vi "I-V.MODEL.vi"(3 "output control":T1, 4 "data":T2, 5 "x":dbl[](array[numeric]), 6 "a":dbl[](array[numeric])) -> (0 "error out":errorcluster, 1 "f'(X,a)":dbl[][](array[numeric]), 2 "f(X, a)":dbl[](array[numeric]))   [LabVIEW 2014]
doc: "This template is the starting point for creating a model function to be passed to the Nonlinear Curve Fit.vi."
uses:
  <vilib>/gmath/NumericalOptimization/objective function data.ctl
  <vilib>/gmath/NumericalOptimization/LM_output select.ctl
  <vilib>/gmath/NI_Gmath.lvlib
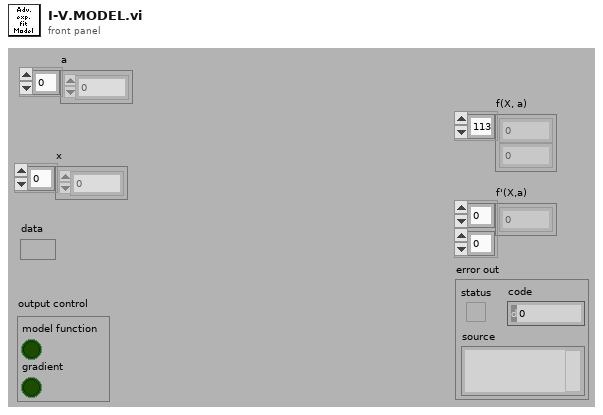
[diagram p1: front panel]
types:
  T1 = typedef "NI_Gmath.lvlib/LM_output select.ctl" = cluster{"model function":bool, "gradient":bool}
  T2 = typedef "NI_Gmath.lvlib/objective function data.ctl" = variant
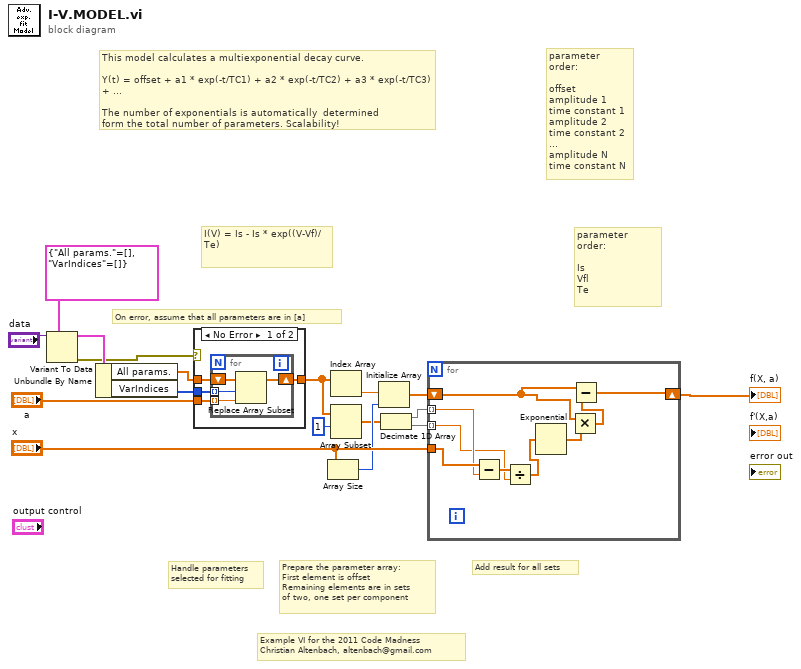
[diagram p0: block diagram]
diagram:
  # "I(V) = Is - Is * exp((V-Vf)/Te)"
  # "parameter order:\n\nIs\nVfl\nTe"
  # "On error, assume that all parameters are in [a]"
  # "This model calculates a multiexponential decay curve.\n\nY(t) = offset + a1 * exp(-t/TC1) + a2 * exp(-t/TC2) + a3 * exp(-t/TC3) + ...\n\nThe number of exponentials is automatically  determined\nform the total number of parameters. Scalability!"
  # "Example VI for the 2011 Code Madness\nChristian Altenbach, altenbach@gmail.com"
  # "Add result for all sets"
  # "Prepare the parameter array:\nFirst element is offset\nRemaining elements are in sets\nof two, one set per component"
  # "Handle parameters\nselected for fitting"
  # "parameter order:\n\noffset\namplitude 1\ntime constant 1\namplitude 2\ntime constant 2\n...\namplitude N\ntime constant N"
  n1 = Variant To Data(type=cluster{"All params.":dbl[], "VarIndices":i32[]} {"All params."=[], "VarIndices"=[]}, Variant="data") -> (data=w7:cluster{"All params.":dbl[], "VarIndices":i32[]}, error out=w1:errorcluster)  [unwired: 1 in]
  n2 = Unbundle By Name(w7) -> ("All params."=w5:dbl[], "VarIndices"=w6:i32[])
  n3 = case shown="No Error" w1 {
    tunnel: "a" -> [w21 w26]
    tunnel: [w20 w26] -> w8
    tunnel: w5 -> [w19 _]
    tunnel: w6 -> [w18 _]
    frame No Error {
      n4 = for {
        shift-right: [w25] -> w20
        shift-left: w19 -> [w24]
        tunnel: w21 -> [w23] mode=indexing
        tunnel: w18 -> [w22] mode=indexing
        n5 = Replace Array Subset(array=w24, new element=w23, index=w22) -> (w25:dbl[])
      }
    }
    frame Error {
    }
  }
  n6 = Array Size(array="x") -> (size(s)=w12:i32)
  n7 = Index Array(array=w8) -> (element=w15:dbl)  [unwired: 1 in]
  n8 = Array Subset(array=w8, index=1) -> (w4:dbl[])  [unwired: 1 in]
  n9 = Initialize Array(w15, w12) -> (w14:dbl[])
  n10 = Decimate 1D Array(w4) -> (w3:dbl[], w2:dbl[])
  n11 = for {
    shift-right: [w27] -> w17
    shift-left: w14 -> [w29]
    tunnel: "x" -> [w34]
    tunnel: w3 -> [w33] mode=indexing
    tunnel: w2 -> [w31] mode=indexing
    n12 = Subtract(x=w34, y=w33) -> (x-y=w32:dbl[])
    n13 = Divide(x=w32, y=w31) -> (x/y=w30:dbl[])
    n14 = Exponential(1:w30) -> (0:w35:dbl[])
    n15 = Multiply(x=w29, y=w35) -> (x*y=w28:dbl[])
    n16 = Subtract(x=w29, y=w28) -> (x-y=w27:dbl[])
  }
  "f(X, a)" <- w17
